vi "ArrayNotesDosMarcoGonzalez.vi"() -> ()   [LabVIEW 2012]
panel:
  out "Array 2":dbl[](array[numeric])
  out "Array":dbl[](array[numeric])
  out "Scalar":dbl
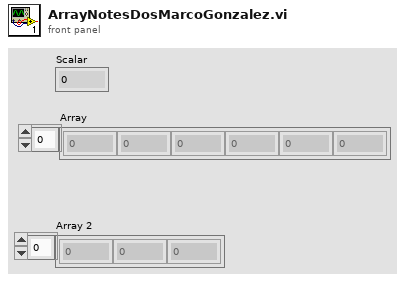
[diagram p1: front panel]
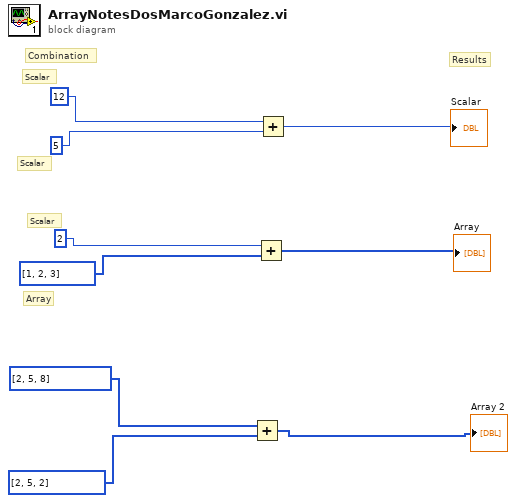
[diagram p0: block diagram]
diagram:
  # "Array"
  # "Scalar"
  # "Scalar"
  # "Scalar"
  # "Results"
  # "Combination"
  n1 = Add(x=i32[] [2, 5, 8], y=i32[] [2, 5, 2]) -> (x+y=→"Array 2":i32[])
  n2 = Add(x=2, y=i32[] [1, 2, 3]) -> (x+y=→"Array":i32[])
  n3 = Add(x=12, y=5) -> (x+y=→"Scalar":i32)
